vi "Error Counter Channel Names.vi"() -> (3 "error counter channel names":string[](array[string]))   [LabVIEW 2020, in "Ballard MIL-STD-1553 Scripting.lvlib"]
uses:
  Ballard MIL-STD-1553 Scripting.lvlib
  Constants.vi
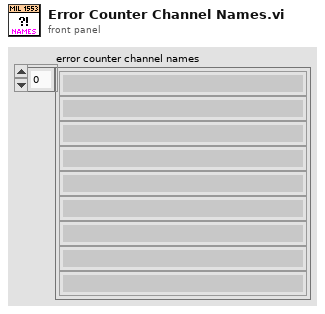
[diagram p1: front panel]
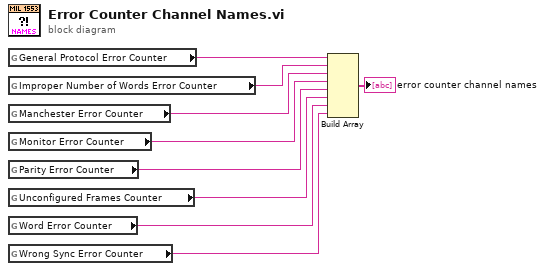
[diagram p0: block diagram]
diagram:
  n1 = global read "Constants.vi" "General Protocol Error Counter"() -> (w2:string)
  n2 = global read "Constants.vi" "Improper Number of Words Error Counter"() -> (w3:string)
  n3 = global read "Constants.vi" "Manchester Error Counter"() -> (w4:string)
  n4 = global read "Constants.vi" "Monitor Error Counter"() -> (w5:string)
  n5 = global read "Constants.vi" "Parity Error Counter"() -> (w6:string)
  n6 = global read "Constants.vi" "Unconfigured Frames Counter"() -> (w7:string)
  n7 = global read "Constants.vi" "Word Error Counter"() -> (w8:string)
  n8 = global read "Constants.vi" "Wrong Sync Error Counter"() -> (w9:string)
  n9 = Build Array(w2, w3, w4, w5, w6, w7, w8, w9) -> (→"error counter channel names":string[])
